vi "get channels.vi"(11 "module configuration in":refnum<class "sample module configuration.lvclass">) -> (2 "channels":refnum<class "TBM channel.lvclass">[](array[class]), 3 "module configuration out":refnum<class "sample module configuration.lvclass">)   [LabVIEW 2013, in "sample module configuration.lvclass"]
uses:
  sample module configuration.lvclass
  channel/TBM channel.lvclass
  sample module configuration.lvclass/sample module configuration.ctl
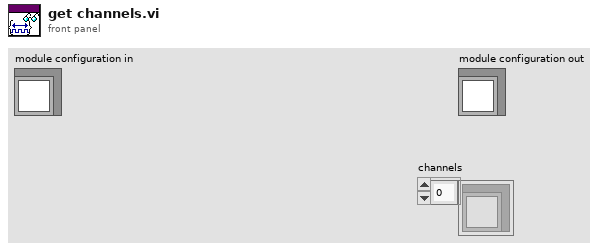
[diagram p1: front panel]
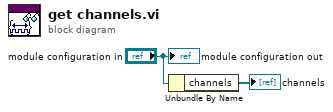
[diagram p0: block diagram]
diagram:
  n1 = Unbundle By Name("module configuration in") -> ("channels"=→"channels":refnum<class "TBM channel.lvclass">[])
  "module configuration out" <- "module configuration in"
